vi "Reserve Network DAQs.vi"() -> ()   [LabVIEW 2020]
uses:
  <vilib>/nisyscfg/nisyscfg.lvlib
  <resource>/objmgr/nicontrollersysapi.rc
  <vilib>/nisyscfg/Close (System).vi
panel:
  out "Progress":i32(slide) scale=0.0..100.0
  out "Name":string
  out "Action":string
  out "close":bool
  in  "Reserve Matched":bool
  in  "Include":bool
  in  "Exclude":bool
  in  "Excluded Devices":i32(listbox)
  in  "Matched Devices":i32(listbox)
  in  "Subnet 4":u8
  in  "Subnet 3":u8=255
  in  "Subnet 2":u8=255
  in  "Subnet 1":u8=255
  in  "Network 4":u8
  in  "Network 3":u8=1
  in  "Network 2":u8=168
  in  "Network 1":u8=192
  # "To exit, click the X"
  # "Match Filter"
  # "Network"
  # "."
  # "."
  # "."
  # "Network Mask"
  # "."
  # "."
  # "."
  # "Double-click to exclude a matched device."
  # "Double-click to remove a device from the exclusion list."
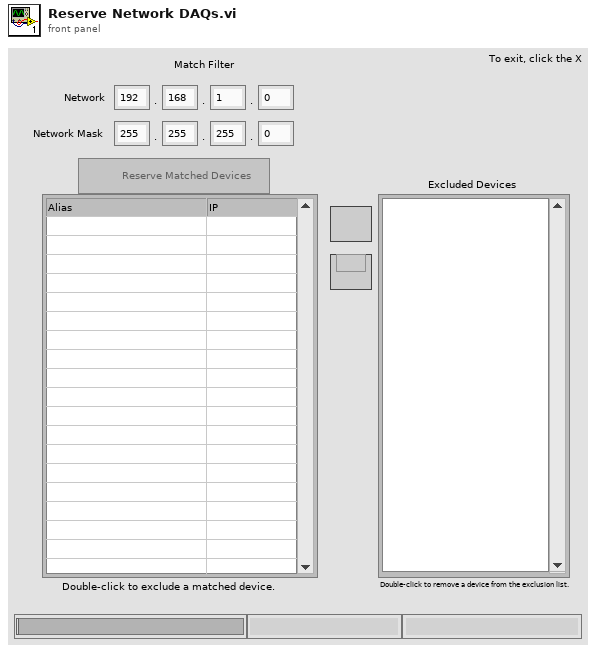
[diagram p1: front panel]
types:
  T1 = enum8{"Enabled", "Disabled", "Disabled and Grayed Out"}
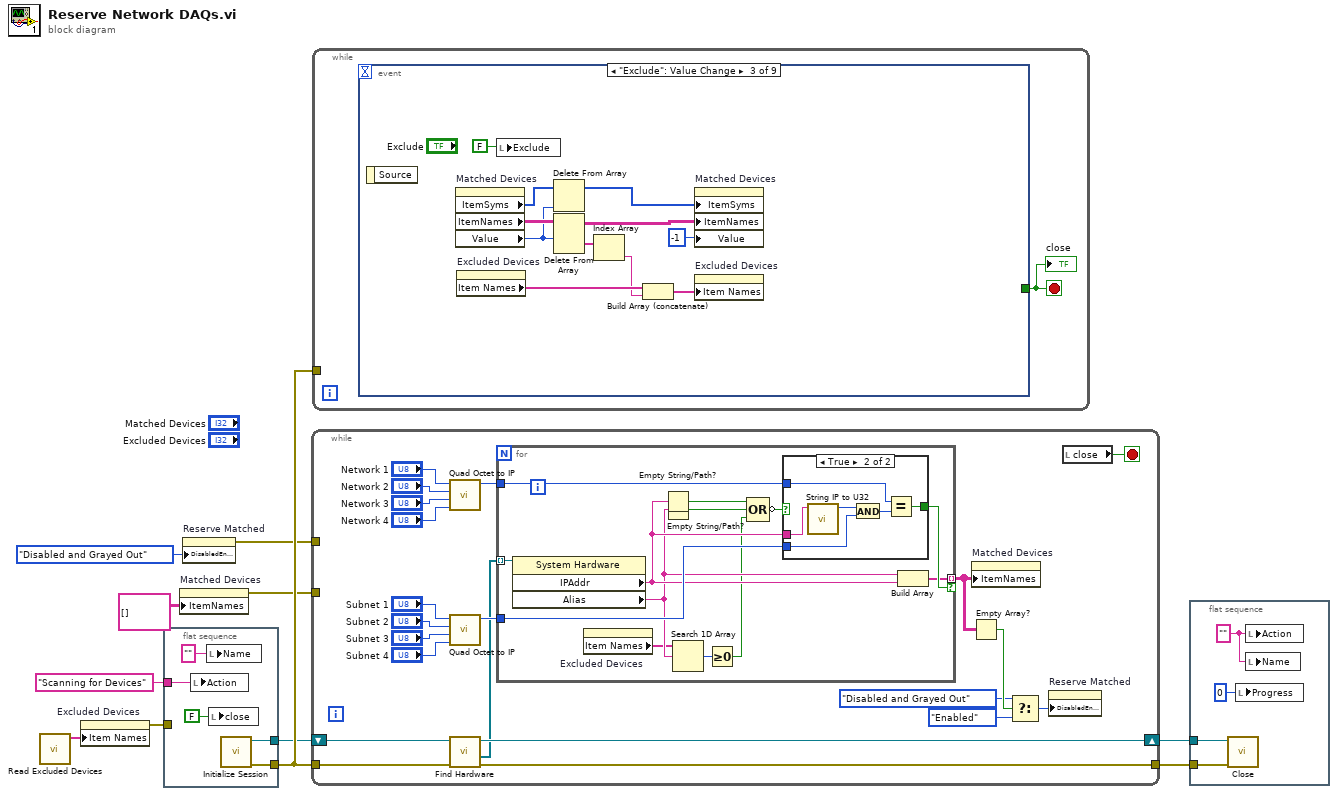
[diagram p0: block diagram]
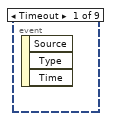
[diagram p3: hidden frame]
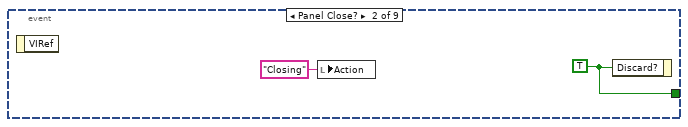
[diagram p4: hidden frame]
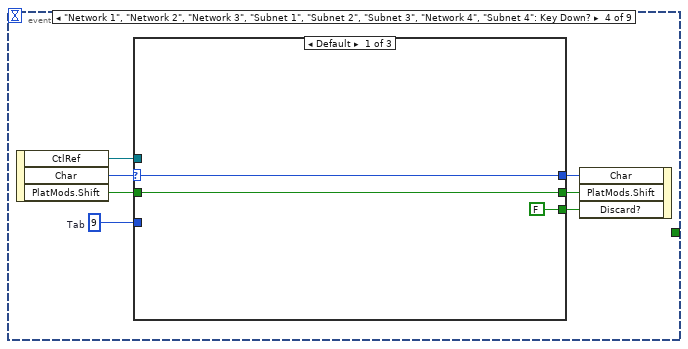
[diagram p5: hidden frame]
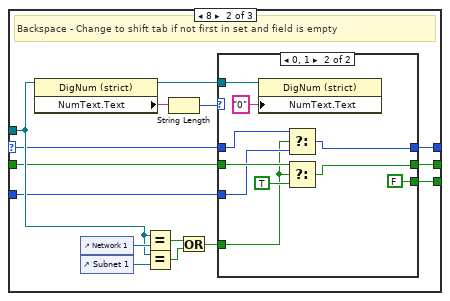
[diagram p6: hidden frame]
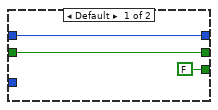
[diagram p7: hidden frame]
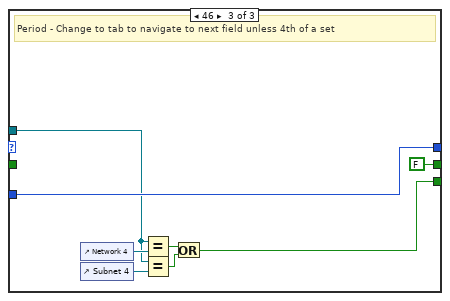
[diagram p8: hidden frame]
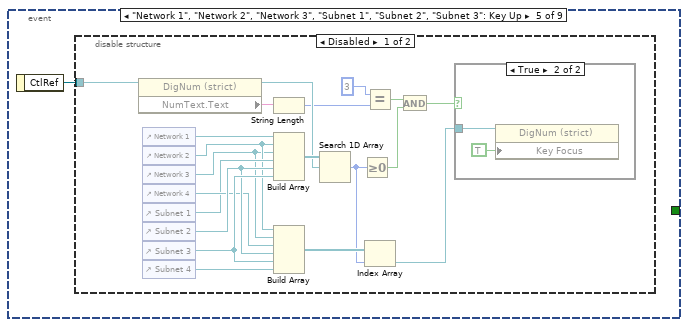
[diagram p9: hidden frame]
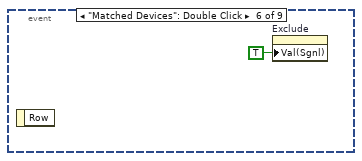
[diagram p12: hidden frame]
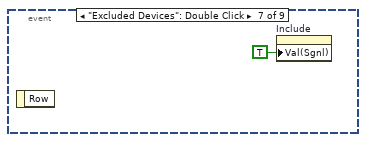
[diagram p13: hidden frame]
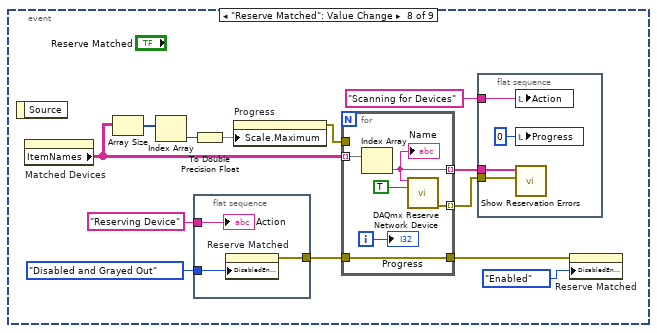
[diagram p14: hidden frame]
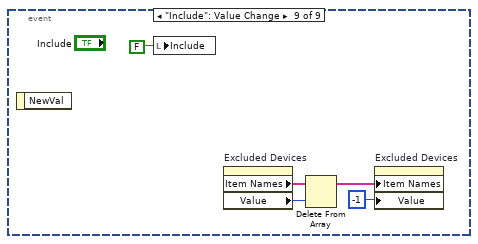
[diagram p15: hidden frame]
diagram:
  n1 = call "Read Excluded Devices.vi"() -> ("Excluded Devices"=w2:string[])  [unwired: 10 in, 1 out]
  n2 = property on="Excluded Devices" class="LstBox (strict)"("Item Names"=w2) -> (error out=w1:errorcluster)  [unwired: 2 in, 1 out]
  n3 = flat-sequence {
    tunnel: [w16] -> w11
    tunnel: [w15] -> w10
    tunnel: "Scanning for Devices" ("Action") -> [w13]
    tunnel: w1 -> [_]
    frame #0 {
      n4 = local write "Action"(w13) -> ()
      n5 = local write "Name"("") -> ()
      n6 = local write "close"(FALSE ("close")) -> ()
      n7 = call <vilib>:"Initialize Session.vi"() -> ("error out"=w16:errorcluster, "Session out"=w15:refnum<k21>)  [unwired: 10 in]
    }
  }
  n8 = property on="Matched Devices" class="MCListbox (strict)"("ItemNames"=string[][] [] ("Item Names")) -> (error out=w4:errorcluster)  [unwired: 2 in, 1 out]
  n9 = property on="Reserve Matched" class="Bool"("DisabledEnum"=T1."Disabled and Grayed Out" ("Disabled")) -> (error out=w5:errorcluster)  [unwired: 2 in, 1 out]
  n10 = while {
    tunnel: w11 -> [w34]
    shift-right: [w36] -> w8
    shift-left: w10 -> [w35]
    tunnel: [w37] -> w9
    tunnel: w5 -> [_]
    tunnel: w4 -> [_]
    stop <- w23 stop-if-true
    n11 = call "Quad Octet to IP.vi"("Octet 4"="Network 4", "Octet 3"="Network 3", "Octet 2"="Network 2", "Octet 1"="Network 1") -> ("U32 IP"=w24:u32)  [unwired: 7 in]
    n12 = call "Quad Octet to IP.vi"("Octet 4"="Subnet 4", "Octet 3"="Subnet 3", "Octet 2"="Subnet 2", "Octet 1"="Subnet 1") -> ("U32 IP"=w25:u32)  [unwired: 7 in]
    n13 = call <vilib>:"Find Hardware.vi"("error in (no error)"=w34, "Session in"=w35) -> ("error out"=w37:errorcluster, "Resources out"=w17:refnum<k20>[], "Session out"=w36:refnum<k21>)  [unwired: 6 in, 1 out]
    n14 = for {
      tunnel: w17 -> [w50] mode=indexing
      tunnel: w25 -> [w49]
      tunnel: w24 -> [w48]
      tunnel: [w45] -> w22 mode=indexing if=w47
      n15 = property class="System Hardware"(reference=w50) -> ("IPAddr"=w46:string, "Alias"=w44:string)  [unwired: 1 in, 2 out]
      n16 = property on="Excluded Devices" class="LstBox (strict)"() -> ("Item Names"=w38:string[])  [unwired: 2 in, 2 out]
      n17 = Empty String/Path?(string/path=w46) -> (empty?=w41:bool)
      n18 = Empty String/Path?(string/path=w44) -> (empty?=w42:bool)
      n19 = Search 1D Array(1D array=w38, element=w44) -> (index of element=w43:i32)  [unwired: 1 in]
      n20 = Greater Or Equal To 0?(x=w43) -> (x >= 0?=w40:bool)
      n21 = Compound Arithmetic op=OR(w41, w42, w40) -> (invert w39:bool)
      n22 = case shown="True" w39 {
        tunnel: w49 -> [_ w55]
        tunnel: w48 -> [_ w54]
        tunnel: [_ w53] -> w47
        tunnel: w46 -> [_ w51]
        frame False {
        }
        frame True {
          n23 = call "String IP to U32.vi"("String IP"=w51) -> ("U32 IP"=w56:u32)  [unwired: 10 in]
          n24 = And(x=w56, y=w55) -> (x .and. y?=w52:u32)
          n25 = Equal?(x=w54, y=w52) -> (x = y?=w53:bool)
        }
      }
      n26 = Build Array(w44, w46) -> (w45:string[])
    }
    n27 = Empty Array?(array=w22) -> (empty?=w21:bool)
    n28 = property on="Matched Devices" class="MCListbox (strict)"("ItemNames"=w22) -> ()  [unwired: 2 in, 2 out]
    n29 = Select(t=T1."Disabled and Grayed Out" ("Disabled"), s=w21, f=T1."Enabled" ("Disabled")) -> (s? t:f=w18:T1)
    n30 = property on="Reserve Matched" class="Bool"("DisabledEnum"=w18) -> ()  [unwired: 2 in, 2 out]
    n31 = local read "close"() -> (w23:bool)
  }
  n32 = while {
    tunnel: w11 -> [_]
    stop <- w57 stop-if-true
    n33 = event shown="[2] \"Exclude\": Value Change" {
      selector: _ -> [_ _ _ _ _ _ _ _ _]
      dyn-events: _ -> [_ _ _ _ _ _ _ _ _]
      timeout: _ -> [_ _ _ _ _ _ _ _ _]
      tunnel: [_ w59 _ _ _ _ _ _ _] -> w57
      event Timeout {
        n34 = event-data() -> ()  [unwired: 1 in, 3 out]
      }
      event Panel Close? {
        w59 = TRUE ("Discard?")
        n35 = event-data() -> ()  [unwired: 1 in, 1 out]
        n36 = local write "Action"("Closing" ("Action")) -> ()
        n37 = event-data("Discard?"=w59) -> ()  [unwired: 1 in, 1 out]
      }
      event "Exclude": Value Change {
        n38 = event-data() -> ()  [unwired: 1 in, 1 out]
        n39 = property on="Matched Devices" class="MCListbox (strict)"() -> ("ItemSyms"=w65:i32[], "ItemNames"=w70:string[][], "Value"=w63:i32)  [unwired: 2 in, 2 out]
        n40 = property on="Excluded Devices" class="LstBox (strict)"() -> ("Item Names"=w67:string[])  [unwired: 2 in, 2 out]
        n41 = local write "Exclude"(FALSE ("Exclude")) -> ()
        n42 = Delete From Array(array=w65, index=w63) -> (array with subset deleted=w64:i32[])  [unwired: 1 in, 1 out]
        n43 = Delete From Array(array=w70, index (row)=w63) -> (deleted portion=w62:string[], array with subset deleted=w69:string[][])  [unwired: 2 in]
        n44 = Index Array(array=w62) -> (element=w61:string)  [unwired: 1 in]
        n45 = Build Array (concatenate)(w67, w61) -> (w66:string[])
        n46 = property on="Matched Devices" class="MCListbox (strict)"("ItemSyms"=w64, "ItemNames"=w69, "Value"=-1 ("Matched Devices")) -> ()  [unwired: 2 in, 2 out]
        n47 = property on="Excluded Devices" class="LstBox (strict)"("Item Names"=w66) -> ()  [unwired: 2 in, 2 out]
      }
      event "Network 1", "Network 2", "Network 3", "Subnet 1", "Subnet 2", "Subnet 3", "Network 4", "Subnet 4": Key Down? {
        w76 = i16 9  # Tab
        n48 = event-data() -> ("CtlRef"=w75:refnum<vi>, "Char"=w77:i16, "PlatMods.Shift"=w74:bool)  [unwired: 1 in]
        n49 = case shown="Default" w77 {
          selector: w77 -> [w80 w90 _]
          tunnel: w76 -> [_ w82 w115]
          tunnel: w75 -> [_ w91 w112]
          tunnel: w74 -> [w79 w88 _]
          tunnel: [w80 w89 w115] -> w73
          tunnel: [w79 w87 FALSE ("Shift")] -> w72
          tunnel: [FALSE w86 w109] -> w71
          frame Default {
          }
          frame 8 {
            # "Backspace - Change to shift tab if not first in set and field is empty"
            n50 = property class="DigNum (strict)"(reference=w91) -> (reference out=w81:refnum<vi>, "NumText.Text"=w85:string)  [unwired: 1 in, 1 out]
            n51 = control-ref of="Network 1"() -> (w95:refnum<vi>)
            n52 = control-ref of="Subnet 1"() -> (w94:refnum<vi>)
            n53 = Equal?(x=w91, y=w95) -> (x = y?=w93:bool)
            n54 = Equal?(x=w91, y=w94) -> (x = y?=w92:bool)
            n55 = String Length(string=w85) -> (length=w84:i32)
            n56 = Or(x=w93, y=w92) -> (x .or. y?=w83:bool)
            n57 = case shown="0, 1" w84 {
              tunnel: w90 -> [w98 w105]
              tunnel: [w98 w103] -> w89
              tunnel: w88 -> [w96 w107]
              tunnel: [w96 w102] -> w87
              tunnel: [FALSE FALSE] -> w86
              tunnel: w83 -> [_ w101]
              tunnel: w82 -> [_ w104]
              tunnel: w81 -> [_ w100]
              frame Default {
              }
              frame 0, 1 {
                n58 = property class="DigNum (strict)"(reference=w100, "NumText.Text"="0" ("Numeric Text.Text")) -> ()  [unwired: 1 in, 2 out]
                n59 = Select(t=w105, s=w101, f=w104) -> (s? t:f=w103:i16)
                n60 = Select(t=w107, s=w101, f=TRUE) -> (s? t:f=w102:bool)
              }
            }
          }
          frame 46 {
            # "Period - Change to tab to navigate to next field unless 4th of a set"
            n61 = control-ref of="Network 4"() -> (w114:refnum<vi>)
            n62 = control-ref of="Subnet 4"() -> (w113:refnum<vi>)
            n63 = Equal?(x=w112, y=w114) -> (x = y?=w111:bool)
            n64 = Equal?(x=w112, y=w113) -> (x = y?=w110:bool)
            n65 = Or(x=w111, y=w110) -> (x .or. y?=w109:bool)
          }
        }
        n66 = event-data("Char"=w73, "PlatMods.Shift"=w72, "Discard?"=w71) -> ()  [unwired: 1 in, 1 out]
      }
      event "Network 1", "Network 2", "Network 3", "Subnet 1", "Subnet 2", "Subnet 3": Key Up {
        n67 = event-data() -> ("CtlRef"=w117:refnum<vi>)  [unwired: 1 in]
        n68 = disable-structure shown="Disabled" {
          disable-tunnel: w117 -> [w130 _]
          frame Disabled {
            n69 = property class="DigNum (strict)"(reference=w130) -> (reference out=w129:refnum<vi>, "NumText.Text"=w127:string)  [unwired: 1 in, 1 out]
            n70 = control-ref of="Network 1"() -> (w137:refnum<vi>)
            n71 = control-ref of="Network 2"() -> (w119:refnum<vi>)
            n72 = control-ref of="Network 3"() -> (w118:refnum<vi>)
            n73 = control-ref of="Network 4"() -> (w133:refnum<vi>)
            n74 = control-ref of="Subnet 1"() -> (w132:refnum<vi>)
            n75 = control-ref of="Subnet 2"() -> (w134:refnum<vi>)
            n76 = control-ref of="Subnet 3"() -> (w135:refnum<vi>)
            n77 = control-ref of="Subnet 4"() -> (w136:refnum<vi>)
            n78 = String Length(string=w127) -> (length=w124:i32)
            n79 = Build Array(w137, w119, w118, w132, w134, w135) -> (w131:refnum<vi>[])
            n80 = Build Array(w119, w118, w133, w134, w135, w136) -> (w128:refnum<vi>[])
            n81 = Search 1D Array(1D array=w131, element=w129) -> (index of element=w125:i32)  [unwired: 1 in]
            n82 = Greater Or Equal To 0?(x=w125) -> (x >= 0?=w121:bool)
            n83 = Equal?(x=3, y=w124) -> (x = y?=w122:bool)
            n84 = Index Array(array=w128, index=w125) -> (element=w126:refnum<vi>)
            n85 = And(x=w122, y=w121) -> (x .and. y?=w120:bool)
            n86 = case shown="True" w120 {
              tunnel: w126 -> [_ w139]
              frame False {
              }
              frame True {
                n87 = property class="DigNum (strict)"(reference=w139, "Key Focus"=TRUE) -> ()  [unwired: 1 in, 2 out]
              }
            }
          }
          frame Enabled {
          }
        }
      }
      event "Matched Devices": Double Click {
        n88 = event-data() -> ()  [unwired: 1 in, 1 out]
        n89 = property on="Exclude" class="Bool (strict)"("Val(Sgnl)"=TRUE ("Value (Signaling)")) -> ()  [unwired: 2 in, 2 out]
      }
      event "Excluded Devices": Double Click {
        n90 = event-data() -> ()  [unwired: 1 in, 1 out]
        n91 = property on="Include" class="Bool (strict)"("Val(Sgnl)"=TRUE ("Value (Signaling)")) -> ()  [unwired: 2 in, 2 out]
      }
      event "Reserve Matched": Value Change {
        n92 = event-data() -> ()  [unwired: 1 in, 1 out]
        n93 = property on="Matched Devices" class="MCListbox (strict)"() -> ("ItemNames"=w147:string[][])  [unwired: 2 in, 2 out]
        n94 = Array Size(array=w147) -> (size(s)=w146:i32[])
        n95 = Index Array(array=w146) -> (element=w145:i32)  [unwired: 1 in]
        n96 = flat-sequence {
          tunnel: T1."Disabled and Grayed Out" ("Disabled") -> [w157]
          tunnel: [w156] -> w153
          tunnel: "Reserving Device" ("Action") -> [w155]
          frame #0 {
            n97 = property on="Reserve Matched" class="Bool"("DisabledEnum"=w157) -> (error out=w156:errorcluster)  [unwired: 2 in, 1 out]
            "Action" <- w155
          }
        }
        n98 = To Double Precision Float(number=w145) -> (double precision float=w144:dbl)
        n99 = property on="Progress" class="Slide (strict)"("Scale.Maximum"=w144) -> (error out=w143:errorcluster)  [unwired: 2 in, 1 out]
        n100 = for {
          tunnel: w147 -> [w167] mode=indexing
          tunnel: w153 -> [w165]
          tunnel: [w165] -> w152
          tunnel: [w164] -> w149 mode=indexing
          tunnel: [w163] -> w150 mode=indexing
          tunnel: w143 -> [_]
          i -> [w162]
          n101 = Index Array(array=w167) -> (element=w163:string)  [unwired: 1 in]
          "Name" <- w163
          n102 = call <vilib>:"DAQmx Reserve Network Device.vi"("device in"=w163, "override reservation?"=TRUE) -> ("error out"=w164:errorcluster)  [unwired: 12 in, 1 out]
          "Progress" <- w162
        }
        n103 = flat-sequence {
          tunnel: w150 -> [w161]
          tunnel: w149 -> [w160]
          tunnel: "Scanning for Devices" ("Action") -> [w158]
          frame #0 {
            n104 = local write "Action"(w158) -> ()
            n105 = local write "Progress"(0 ("Progress")) -> ()
            n106 = call "Show Reservation Errors.vi"("Errors"=w160, "Aliases"=w161) -> ()  [unwired: 10 in]
          }
        }
        n107 = property on="Reserve Matched" class="Bool"(error in=w152, "DisabledEnum"=T1."Enabled" ("Disabled")) -> ()  [unwired: 1 in, 2 out]
      }
      event "Include": Value Change {
        n108 = event-data() -> ()  [unwired: 1 in, 1 out]
        n109 = local write "Include"(FALSE ("Include")) -> ()
        n110 = property on="Excluded Devices" class="LstBox (strict)"() -> ("Item Names"=w171:string[], "Value"=w170:i32)  [unwired: 2 in, 2 out]
        n111 = Delete From Array(array=w171, index=w170) -> (array with subset deleted=w169:string[])  [unwired: 1 in, 1 out]
        n112 = property on="Excluded Devices" class="LstBox (strict)"("Item Names"=w169, "Value"=-1 ("Excluded Devices")) -> ()  [unwired: 2 in, 2 out]
      }
    }
    "close" <- w57
  }
  n113 = flat-sequence {
    tunnel: w9 -> [w176]
    tunnel: w8 -> [w175]
    frame #0 {
      w174 = ""
      n114 = call-poly <vilib>:"Close.vi"("error in (no error)"=w176, "Session in"=w175) -> ()  [unwired: 9 in, 1 out]
      n115 = local write "Progress"(0 ("Progress")) -> ()
      n116 = local write "Action"(w174) -> ()
      n117 = local write "Name"(w174) -> ()
    }
  }
